vi "PDC_GetHeadTypeName.vi"(8 "error in (no error)":errorcluster, 9 "HeadNo":u32, 10 "ChildNo":u32, 11 "DeviceNo":u32) -> (0 "error out":errorcluster, 2 "StrName":string, 3 "ReturnValue":u32, 4 "ErrorCode":u32)   [LabVIEW 8.6]
doc: "Retrives a head type name of specified child deviece."
uses:
  sub/global.vi
  PDCLIB.dll
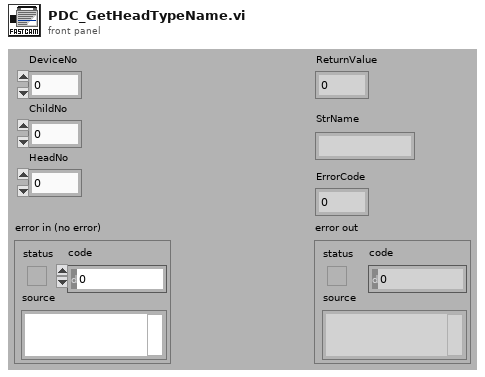
[diagram p1: front panel]
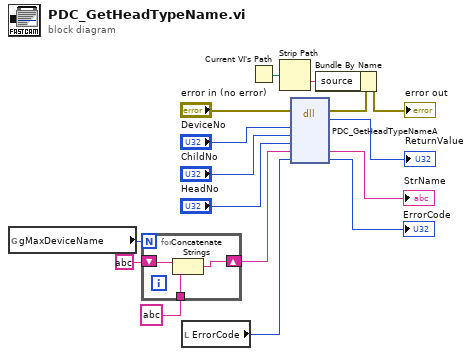
[diagram p0: block diagram]
diagram:
  n1 = global read "global.vi" "gMaxDeviceName"() -> (w6:i32)
  n2 = for {
    N: w6 -> [_]
    shift-right: [w19] -> w7
    shift-left: string ? -> [w18]
    tunnel: string ? -> [w17]
    n3 = Concatenate Strings(w18, w17) -> (w19:string)
  }
  n4 = local read "ErrorCode"() -> (w13:u32)
  n5 = Current VI's Path() -> (path=w3:path)
  n6 = Strip Path(path=w3) -> (name=w4:string)  [unwired: 1 out]
  n7 = dll-call lib="PDCLIB.dll" fn="PDC_GetHeadTypeNameA"(error in="error in (no error)", "nDeviceNo"="DeviceNo", "nChildNo"="ChildNo", "nHeadNo"="HeadNo", "pStrName"=w7, "pErrorCode"=w13) -> (error out=w2:errorcluster, "return type"=→"ReturnValue":u32, "pStrName"=→"StrName":string, "pErrorCode"=→"ErrorCode":u32)  [unwired: 5 in, 1 out]
  n8 = Bundle By Name(cluster=w2, "source"=w4) -> (→"error out":errorcluster)
